vi "Pad-And-Convert.vi"(11 "Array in":u8[](array[numeric])=[16, 1, 10, 0, 1, 100, 137, 240, 0, 0, 0, 0, 0, 0, 0, 0, 0, 12, 1, 2, 3, 4, 5, 6, 7, 8, 9, 10, 112] format="%.0x") -> (3 "Array":u32[](array[numeric])=[655632, 4035535873, 0, 0, 33623040, 100992003, 168364039, 1879048192] format="%.0x")   [LabVIEW 2018]
panel:
  out "y":u32=112 format="%.0x"
  out "Array 3":u32[](array[numeric])=[112] format="%.0x"
  out "Array 2":u32[](array[numeric])=[112] format="%.0x"
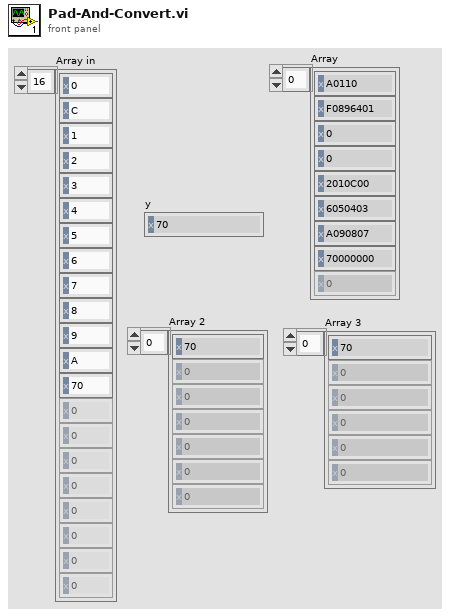
[diagram p1: front panel]
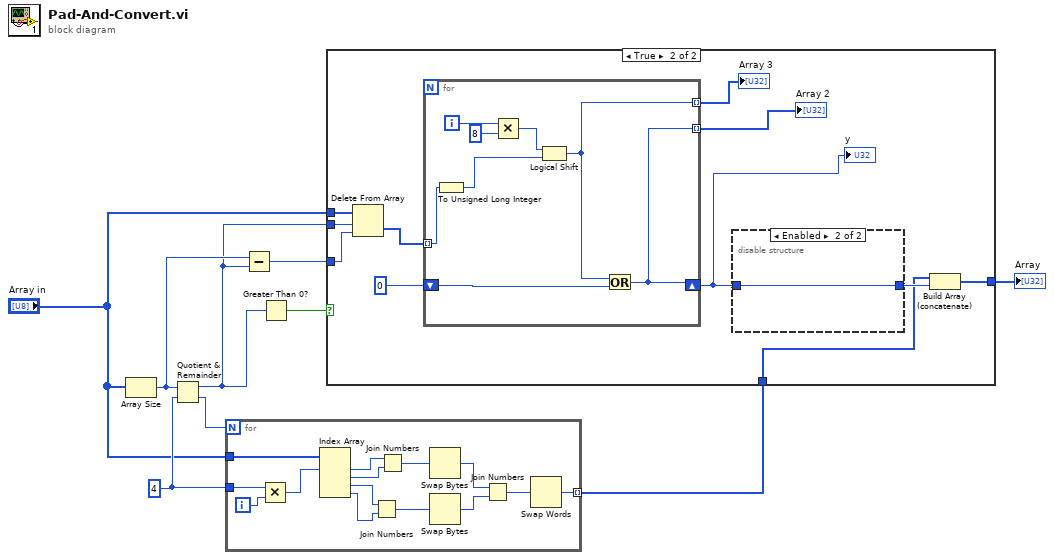
[diagram p0: block diagram]
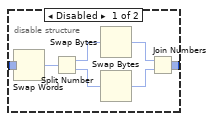
[diagram p3: hidden frame]
diagram:
  w8 = 4 ("y")
  n1 = Array Size(array="Array in") -> (size(s)=w4:i32)
  n2 = Quotient & Remainder(x=w4, y=w8) -> (x-y*floor(x/y)=w3:i32, floor(x/y)=w9:i32)
  n3 = for {
    N: w9 -> [_]
    tunnel: w8 -> [w22]
    tunnel: "Array in" -> [w21]
    tunnel: [w10] -> w7 mode=indexing
    i -> [w23]
    n4 = Multiply(x=w22, y=w23) -> (x*y=w20:i32)
    n5 = Index Array(array=w21, index #1=w20) -> (element #1=w19:u8, element #2=w16:u8, element #3=w17:u8, element #4=w18:u8)  [unwired: 3 in]
    n6 = Join Numbers(hi=w17, lo=w18) -> ((hi.lo)=w12:u16)
    n7 = Join Numbers(hi=w19, lo=w16) -> ((hi.lo)=w14:u16)
    n8 = Swap Bytes(anything=w14) -> (byte swapped=w13:u16)
    n9 = Swap Bytes(anything=w12) -> (byte swapped=w11:u16)
    n10 = Join Numbers(hi=w13, lo=w11) -> ((hi.lo)=w15:u32)
    n11 = Swap Words(1:w15) -> (0:w10:u32)
  }
  n12 = Subtract(x=w4, y=w3) -> (x-y=w5:i32)
  n13 = Greater Than 0?(x=w3) -> (x > 0?=w1:bool)
  n14 = case shown="True" w1 {
    tunnel: w7 -> [w24 w28]
    tunnel: [w24 w35] -> w6
    tunnel: w5 -> [_ w34]
    tunnel: w3 -> [_ w33]
    tunnel: "Array in" -> [_ w32]
    frame False {
    }
    frame True {
      n15 = Delete From Array(array=w32, length=w33, index=w34) -> (deleted portion=w30:u8[])  [unwired: 1 out]
      n16 = for {
        shift-right: [w45] -> w27
        shift-left: u32 0 ("y") -> [w51]
        tunnel: w30 -> [w50] mode=indexing
        tunnel: [w45] -> w26 mode=indexing
        tunnel: [w44] -> w25 mode=indexing
        i -> [w49]
        n17 = To Unsigned Long Integer(number=w50) -> (unsigned 32bit integer=w46:u32)
        n18 = Multiply(x=w49, y=8) -> (x*y=w47:i32)
        n19 = Logical Shift(y=w47, x=w46) -> (x << y=w44:u32)
        n20 = Or(x=w44, y=w51) -> (x .or. y?=w45:u32)
      }
      "Array 2" <- w26
      "Array 3" <- w25
      "y" <- w27
      n21 = disable-structure shown="Enabled" {
        disable-tunnel: [w41 w43] -> w29
        disable-tunnel: w27 -> [w36 w43]
        frame Disabled {
          n22 = Swap Words(1:w36) -> (0:w42:u32)
          n23 = Split Number(x=w42) -> (hi(x)=w39:u16, lo(x)=w40:u16)
          n24 = Swap Bytes(anything=w39) -> (byte swapped=w38:u16)
          n25 = Swap Bytes(anything=w40) -> (byte swapped=w37:u16)
          n26 = Join Numbers(hi=w38, lo=w37) -> ((hi.lo)=w41:u32)
        }
        frame Enabled {
        }
      }
      n27 = Build Array (concatenate)(w28, w29) -> (w35:u32[])
    }
  }
  "Array" <- w6
